vi "Read 00-00-9220.vi"() -> (3 "00-00-9220":dbl[](array[numeric]))   [LabVIEW 2018]
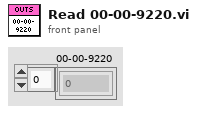
[diagram p1: front panel]
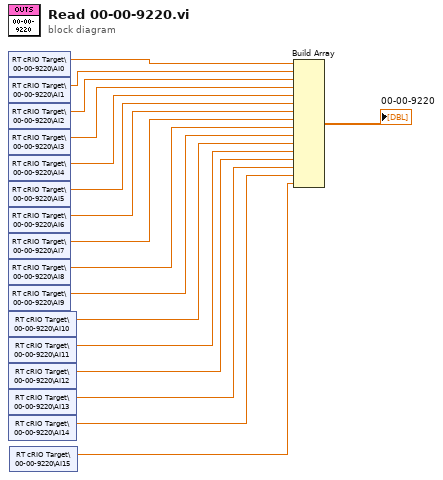
[diagram p0: block diagram]
diagram:
  n1 = shared-variable "RT cRIO Target\\00-00-9220\\AI0"() -> (w1:dbl)  [unwired: 1 in, 1 out]
  n2 = shared-variable "RT cRIO Target\\00-00-9220\\AI1"() -> (w2:dbl)  [unwired: 1 in, 1 out]
  n3 = shared-variable "RT cRIO Target\\00-00-9220\\AI2"() -> (w3:dbl)  [unwired: 1 in, 1 out]
  n4 = shared-variable "RT cRIO Target\\00-00-9220\\AI3"() -> (w4:dbl)  [unwired: 1 in, 1 out]
  n5 = shared-variable "RT cRIO Target\\00-00-9220\\AI4"() -> (w5:dbl)  [unwired: 1 in, 1 out]
  n6 = shared-variable "RT cRIO Target\\00-00-9220\\AI5"() -> (w6:dbl)  [unwired: 1 in, 1 out]
  n7 = shared-variable "RT cRIO Target\\00-00-9220\\AI6"() -> (w7:dbl)  [unwired: 1 in, 1 out]
  n8 = shared-variable "RT cRIO Target\\00-00-9220\\AI7"() -> (w8:dbl)  [unwired: 1 in, 1 out]
  n9 = shared-variable "RT cRIO Target\\00-00-9220\\AI8"() -> (w9:dbl)  [unwired: 1 in, 1 out]
  n10 = shared-variable "RT cRIO Target\\00-00-9220\\AI9"() -> (w10:dbl)  [unwired: 1 in, 1 out]
  n11 = shared-variable "RT cRIO Target\\00-00-9220\\AI10"() -> (w11:dbl)  [unwired: 1 in, 1 out]
  n12 = shared-variable "RT cRIO Target\\00-00-9220\\AI11"() -> (w12:dbl)  [unwired: 1 in, 1 out]
  n13 = shared-variable "RT cRIO Target\\00-00-9220\\AI12"() -> (w13:dbl)  [unwired: 1 in, 1 out]
  n14 = shared-variable "RT cRIO Target\\00-00-9220\\AI13"() -> (w14:dbl)  [unwired: 1 in, 1 out]
  n15 = shared-variable "RT cRIO Target\\00-00-9220\\AI14"() -> (w15:dbl)  [unwired: 1 in, 1 out]
  n16 = shared-variable "RT cRIO Target\\00-00-9220\\AI15"() -> (w16:dbl)  [unwired: 1 in, 1 out]
  n17 = Build Array(w1, w2, w3, w4, w5, w6, w7, w8, w9, w10, w11, w12, w13, w14, w15, w16) -> (→"00-00-9220":dbl[])
